vi "GetCurrentPath.vi"(8 "Error In":errorcluster) -> (0 "Error Out":errorcluster, 3 "Current VI Path Out":path)   [LabVIEW 2011]
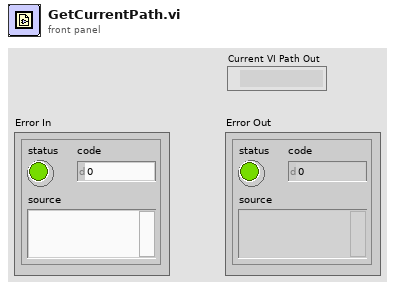
[diagram p1: front panel]
types:
  T1 = enum32{"invalid app kind", "Development System", "Run Time System", "Student Edition", "Embedded LabVIEW", "Evaluation", "Custom"}
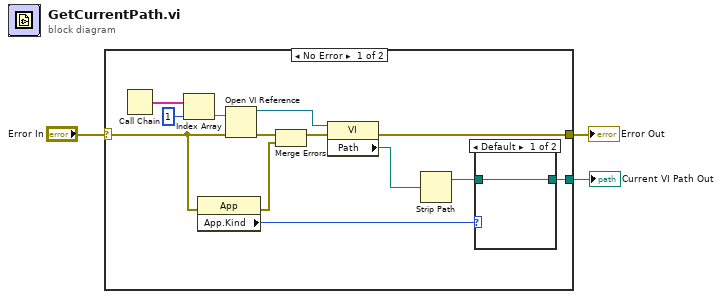
[diagram p0: block diagram]
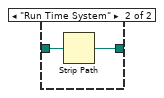
[diagram p2: hidden frame]
diagram:
  n1 = case shown="No Error" "Error In" {
    selector: "Error In" -> [w5 w20]
    tunnel: [w11 w20] -> w3
    tunnel: [w6 _] -> w2
    frame No Error {
      n2 = Call Chain() -> (call chain=w16:string[])
      n3 = Index Array(array=w16, index=1) -> (element=w15:string)
      n4 = property class="App"(error in=w5) -> (error out=w9:errorcluster, "App.Kind"=w10:T1)  [unwired: 1 in, 1 out]
      n5 = Open VI Reference(vi path=w15, error in (no error)=w5) -> (vi reference=w14:refnum<vi>, error out=w8:errorcluster)  [unwired: 4 in]
      n6 = Merge Errors(w8, w9) -> (w7:errorcluster)
      n7 = property class="VI"(reference=w14, error in=w7) -> (error out=w11:errorcluster, "Path"=w13:path)  [unwired: 1 out]
      n8 = Strip Path(path=w13) -> (stripped path=w12:path)  [unwired: 1 out]
      n9 = case shown="Default" w10 {
        tunnel: w12 -> [w17 w19]
        tunnel: [w17 w18] -> w6
        frame Default {
        }
        frame "Run Time System" {
          n10 = Strip Path(path=w19) -> (stripped path=w18:path)  [unwired: 1 out]
        }
      }
    }
    frame Error {
    }
  }
  "Error Out" <- w3
  "Current VI Path Out" <- w2
